vi "sta_std and variance (SubVI).vi"(5 "array":dbl[](array[numeric]), 11 "에러 입력(에러 없음)":errorcluster) -> (4 "참조 번호 출력":refnum<k35>, 6 "mean":dbl, 8 "standard deviation":dbl, 10 "variance":dbl, 15 "에러 출력":errorcluster)   [LabVIEW 2018]
uses:
  PythonConfigGlobal.vi
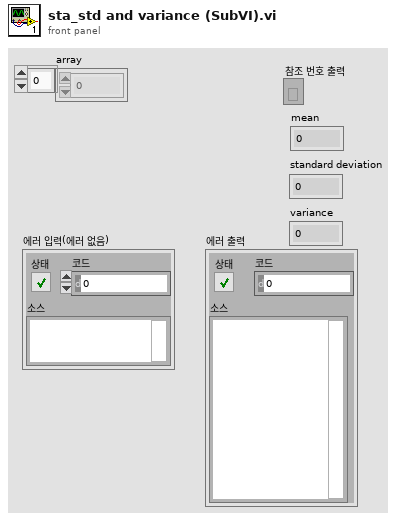
[diagram p1: front panel]
types:
  T1 = cluster{"session out":refnum<k35>, "appended path":path}
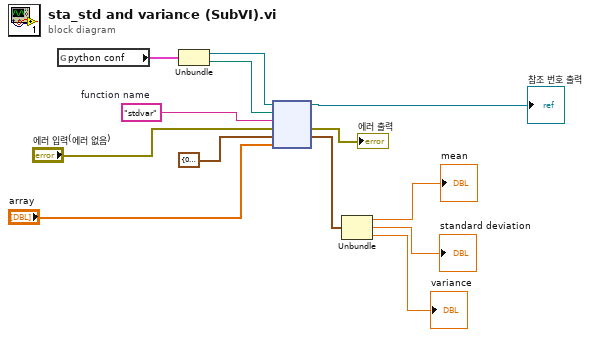
[diagram p0: block diagram]
diagram:
  w2 = "stdvar"  # function name
  n1 = global read "PythonConfigGlobal.vi" "python conf"() -> (w7:T1)
  n2 = Unbundle(w7) -> ("session out"=w3:refnum<k35>, "appended path"=w4:path)
  n3 = node(w3, w4, w2, "에러 입력(에러 없음)", cluster{"mean":dbl, "std":dbl, "var":dbl} {"mean"=0.0, "std"=0.0, "var"=0.0}, "array") -> (→"참조 번호 출력":refnum<k35>, →"에러 출력":errorcluster, w1:cluster{"mean":dbl, "std":dbl, "var":dbl})  [unwired: 1 in, 2 out]
  n4 = Unbundle(w1) -> ("mean"=→"mean":dbl, "std"=→"standard deviation":dbl, "var"=→"variance":dbl)
